vi "10.3.vi"() -> ()   [LabVIEW 2012]
panel:
  out "DAC Deviation":cluster{"Y":dbl[], "Y":dbl[]}[](graph)
  out "DAC Output":cluster{"Y":dbl[], "Y":dbl[]}[](graph)
  out "Actual DAC Output":dbl
  out "Desired DAC Output":dbl
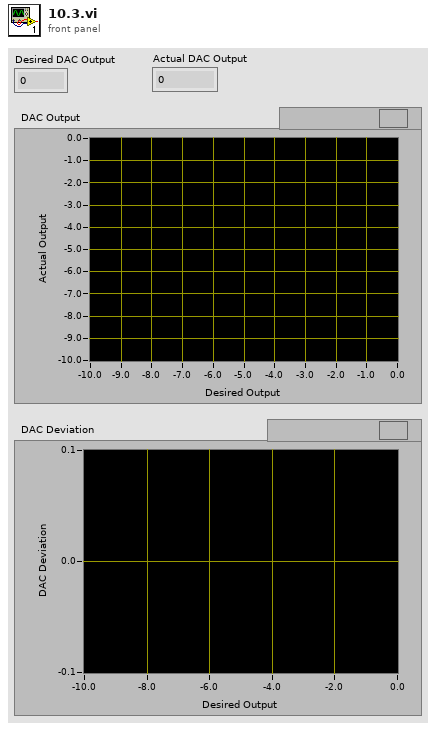
[diagram p1: front panel]
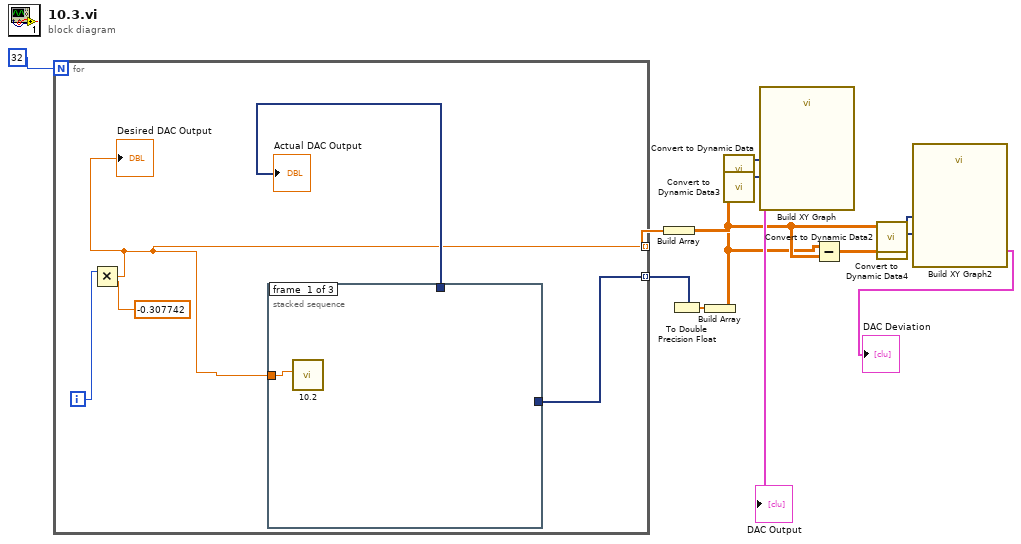
[diagram p0: block diagram]
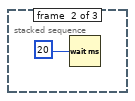
[diagram p2: hidden frame]
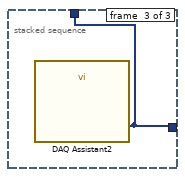
[diagram p3: hidden frame]
diagram:
  n1 = for {
    N: 32 -> [_]
    tunnel: [w15] -> w10 mode=indexing
    tunnel: [w14] -> w9 mode=indexing
    i -> [w17]
    n2 = Multiply(x=w17, y=-0.307742) -> (x*y=w15:dbl)
    "Desired DAC Output" <- w15
    n3 = stacked-sequence {
      tunnel: w15 -> [w19 _ _]
      tunnel: [_ _ w21] -> w16
      tunnel: [_ _ w21] -> w14
      frame #0 {
        n4 = call "10.2.vi"("DAC Output Voltage"=w19) -> ()  [unwired: 11 in]
      }
      frame #1 {
        n5 = Wait (ms)(milliseconds to wait=u32 20) -> ()  [unwired: 1 out]
      }
      frame #2 {
        n6 = call "DAQ Assistant2"() -> ("data"=w21:dynamicdata)  [unwired: 17 in, 2 out]
      }
    }
    "Actual DAC Output" <- w16
  }
  n7 = Build Array(w10) -> (w4:dbl[][])
  n8 = To Double Precision Float(number=w9) -> (double precision float=w7:dbl[])
  n9 = Build Array(w7) -> (w3:dbl[][])
  n10 = call "Convert to Dynamic Data"("2D Array"=w4) -> ("Dynamic Data Type"=w6:dynamicdata)  [unwired: 3 in]
  n11 = call "Convert to Dynamic Data3"("2D Array"=w3) -> ("Dynamic Data Type"=w8:dynamicdata)  [unwired: 3 in]
  n12 = call "Build XY Graph"("Y Input"=w8, "X Input"=w6) -> ("XY Graph"=→"DAC Output":cluster{"Y":dbl[], "Y":dbl[]}[])  [unwired: 3 in, 6 out]
  n13 = Subtract(x=w3, y=w4) -> (x-y=w2:dbl[][])
  n14 = call "Convert to Dynamic Data2"("2D Array"=w4) -> ("Dynamic Data Type"=w5:dynamicdata)  [unwired: 3 in]
  n15 = call "Convert to Dynamic Data4"("2D Array"=w2) -> ("Dynamic Data Type"=w1:dynamicdata)  [unwired: 3 in]
  n16 = call "Build XY Graph2"("Y Input"=w1, "X Input"=w5) -> ("XY Graph"=→"DAC Deviation":cluster{"Y":dbl[], "Y":dbl[]}[])  [unwired: 3 in, 6 out]
